vi "Ini.vi"(8 "error in":errorcluster, 10 "IP section":string="Modbus", 11 "INI file path":path=path "C:/Users/User/Desktop/YDX701_TDC/iniData/TDC_IniData.ini") -> (0 "Kollmorgan":string, 1 "PLC":string, 2 "TCP2Foxc":string, 3 "SR1000":string)   [LabVIEW 2019]
uses:
  <vilib>/Utility/config.llb/Read Key (String).vi
  <vilib>/Utility/config.llb/NI_LVConfig.lvlib
panel:
  out "error out":errorcluster
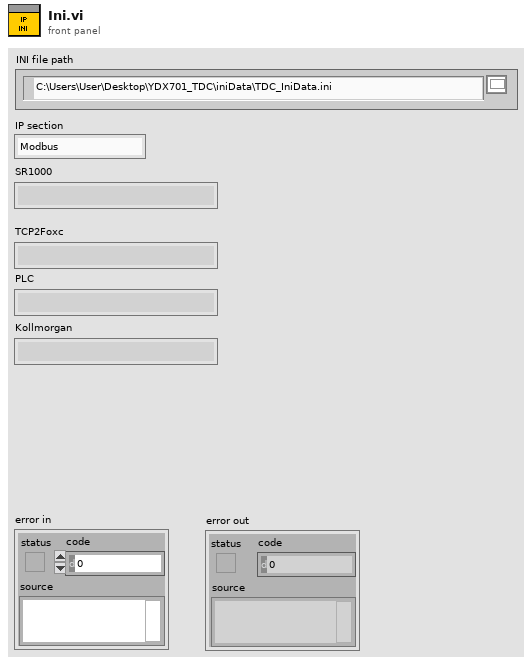
[diagram p1: front panel]
types:
  T1 = typedef "NI_LVConfig.lvlib/Config Data RefNum.ctl" = refnum<k1>
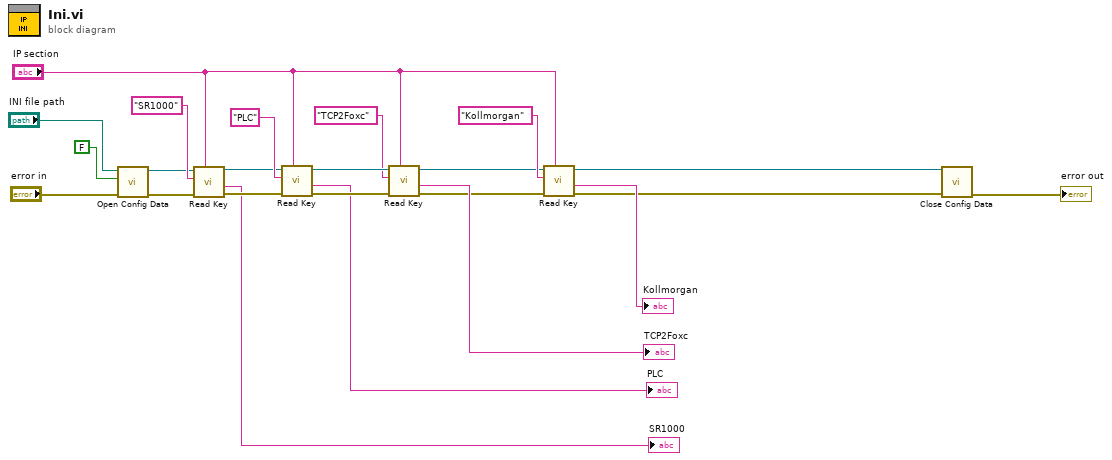
[diagram p0: block diagram]
diagram:
  n1 = call <vilib>:"Open Config Data.vi"("error in (no error)"="error in", "create file if necessary (T)"=FALSE ("create file if necessary? (T)"), "configuration file path"="INI file path") -> ("error out"=w21:errorcluster, "refnum"=w19:T1)  [unwired: 6 in, 1 out]
  n2 = call-poly <vilib>:"Read Key.vi"("section"="IP section", "error in (no error)"=w21, "key"="SR1000", "refnum"=w19) -> ("error out"=w14:errorcluster, "value"=→"SR1000":string, "refnum out"=w15:T1)  [unwired: 2 in, 3 out]
  n3 = call-poly <vilib>:"Read Key.vi"("section"="IP section", "error in (no error)"=w14, "key"="PLC", "refnum"=w15) -> ("error out"=w11:errorcluster, "value"=→"PLC":string, "refnum out"=w12:T1)  [unwired: 2 in, 3 out]
  n4 = call-poly <vilib>:"Read Key.vi"("section"="IP section", "error in (no error)"=w11, "key"="TCP2Foxc", "refnum"=w12) -> ("error out"=w6:errorcluster, "value"=→"TCP2Foxc":string, "refnum out"=w5:T1)  [unwired: 2 in, 3 out]
  n5 = call-poly <vilib>:"Read Key.vi"("section"="IP section", "error in (no error)"=w6, "key"="Kollmorgan", "refnum"=w5) -> ("error out"=w1:errorcluster, "value"=→"Kollmorgan":string, "refnum out"=w2:T1)  [unwired: 2 in, 3 out]
  n6 = call <vilib>:"Close Config Data.vi"("error in (no error)"=w1, "refnum"=w2) -> ("error out"=→"error out":errorcluster)  [unwired: 1 in, 8 out]
